vi "Teleop.vi"(10 "Match Info":T1={"Autonomous Elapsed Seconds"=0.0, "TeleOp Elapsed Seconds"=0.0, "Disabled Elapsed Seconds"=0.0, "Visited Autonomous"=FALSE, "Visited TeleOp"=FALSE, "Visited Disabled"=FALSE, "Autonomous Settings"={"Autonomous Style"=enum."Independent", "VI Refnum"=refnum}}, 11 "Call Context":T2) -> ()   [LabVIEW 2017]
doc: "This VI is called for each enabled TeleOp packet received from the DS. It is typically used to read from joysticks and other inputs and update I/O or setpoints for timed control loops. It should complete and return within 20 milliseconds or risk missing DS packets."
uses:
  <vilib>/Rock Robotics/WPI/DriverStation/WPI_DriverStationDerivedRobotMode.ctl
  <vilib>/Rock Robotics/WPI/DriverStation/WPI_DriverStationMatch Info.ctl
  <vilib>/Rock Robotics/WPI/Utilities/WPI_GetSetVariantRefNum.vi
  <vilib>/Rock Robotics/Network Tables/NT Write Boolean Array.vi
  <vilib>/Rock Robotics/Network Tables/NT Write Numeric Array.vi
  Framework/Robot Global Data.vi
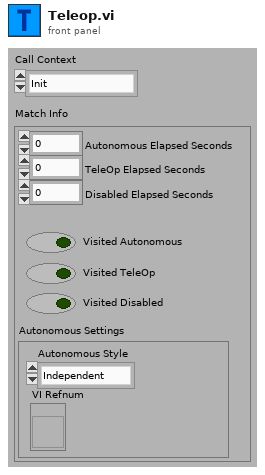
[diagram p1: front panel]
types:
  T1 = typedef "WPI_DriverStationMatch Info.ctl" = cluster{"Autonomous Elapsed Seconds":dbl, "TeleOp Elapsed Seconds":dbl, "Disabled Elapsed Seconds":dbl, "Visited Autonomous":bool, "Visited TeleOp":bool, "Visited Disabled":bool, "Autonomous Settings":cluster{"Autonomous Style":enum16{"Iterative", "Independent"}, "VI Refnum":refnum<vi>}}
  T2 = typedef "WPI_DriverStationDerivedRobotMode.ctl" = enum16{"Init", "Execute", "Stop"}
  T3 = enum16{"Linear", "Square  Root", "Square", "n^x"}
  T4 = typedef "WPI_JoystickDevRef.ctl" = cluster{"Device":T5}
  T5 = typedef "WPI_JoystickDeviceEnum.ctl" = enum16{"USB 0", "USB 1", "USB 2", "USB 3", "USB 4", "USB 5"}
  T6 = cluster{"X":dbl, "Y":dbl, "Angle":dbl, "Magnitude":dbl}
  T7 = typedef "Command Status Info.ctl" = cluster{"Name":string, "Status":T8, "notifier out":T9}
  T8 = typedef "Completion Status.ctl" = enum16{"Successful", "Aborted", "Incomplete"}
  T9 = typedef "Completion Notifier.ctl" = refnum<notifier>
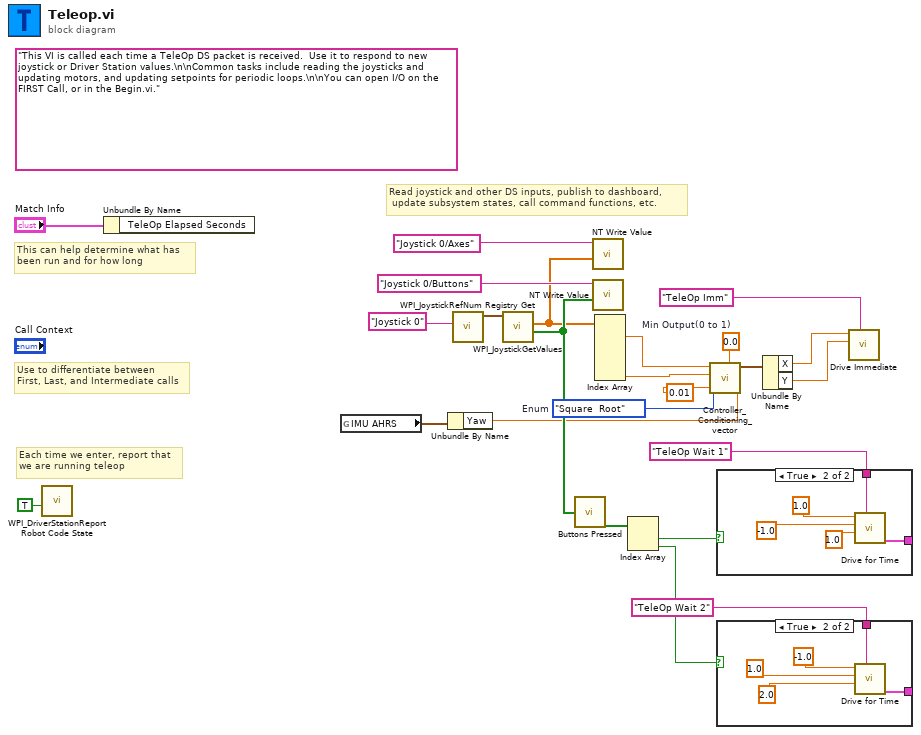
[diagram p0: block diagram]
diagram:
  w4 = T3."Square  Root"  # Enum
  w5 = 0.0  # Min Output(0 to 1)
  (unwired) "This VI is called each time a TeleOp DS packet is received.  Use it to respond to new joystick or Driver Station values.\n\nCommon tasks include reading the joysticks and updating motors, and updating setpoints for periodic loops.\n\nYou can open I/O on the FIRST Call, or in the Begin.vi."
  # "Read joystick and other DS inputs, publish to dashboard,\n update subsystem states, call command functions, etc."
  # "Each time we enter, report that\nwe are running teleop"
  # "Use to differentiate between\nFirst, Last, and Intermediate calls"
  # "This can help determine what has\nbeen run and for how long"
  n1 = call <vilib>:"WPI_DriverStationReport Robot Code State.vi"("TeleOp"=TRUE ("Autonomous")) -> ()  [unwired: 10 in, 1 out]
  n2 = Unbundle By Name("Match Info") -> ()  [unwired: 1 out]
  n3 = global read "Robot Global Data.vi" "IMU AHRS"() -> (w8:cluster{"Pitch":dbl, "Roll":dbl, "Yaw":dbl})
  n4 = Unbundle By Name(w8) -> ("Yaw"=w7:dbl)
  n5 = call <vilib>:"WPI_JoystickRefNum Registry Get.vi"("refnum name"="Joystick 0") -> ("JoystickDevRef"=w21:T4)  [unwired: 1 in, 9 out]
  n6 = call <vilib>:"WPI_JoystickGetValues.vi"("JoystickDevRef"=w21) -> ("Buttons"=w13:bool[], "Axes"=w12:dbl[])  [unwired: 6 in, 3 out]
  n7 = call "Buttons Pressed.vi"("Button Values"=w13) -> ("Button Presses"=w17:bool[])
  n8 = call-poly <vilib>:"NT Write Value.vi"("Numeric Array"=w12, "Name"="Joystick 0/Axes") -> ()  [unwired: 9 in, 1 out]
  n9 = call-poly <vilib>:"NT Write Value.vi"("Boolean Array"=w13, "Name"="Joystick 0/Buttons") -> ()  [unwired: 9 in, 1 out]
  n10 = Index Array(array=w12) -> (element #1=w10:dbl, element #6=w9:dbl)  [unwired: 6 in, 4 out]
  n11 = Index Array(array=w17) -> (element #1=w16:bool, element #2=w15:bool)  [unwired: 2 in]
  n12 = call "Controller_Conditioning_vector.vi"("Angular Offset\n(-180 to 180 or 0 to 360)"=w7, "Min Output(0 to 1)"=w5, "Enum"=w4, "Dead Zone(0 to 1)"=0.01, "Y(-1 to 1)"=w9, "X(-1 to 1)"=w10) -> ("output cluster"=w3:T6)  [unwired: 5 in]
  n13 = case shown="True" w16 {
    tunnel: [_ w28] -> _
    tunnel: "TeleOp Wait 1" ("Description") -> [_ w27]
    frame False {
    }
    frame True {
      n14 = call "Drive for Time.vi"("Description"=w27, "Seconds"=1.0, "Right Speed"=-1.0, "Left Speed"=1.0) -> ("Command Info Out"=w28:T7)  [unwired: 6 in, 1 out]
    }
  }
  n15 = case shown="True" w15 {
    tunnel: [_ w32] -> _
    tunnel: "TeleOp Wait 2" ("Description") -> [_ w31]
    frame False {
    }
    frame True {
      n16 = call "Drive for Time.vi"("Description"=w31, "Seconds"=2.0, "Right Speed"=1.0, "Left Speed"=-1.0) -> ("Command Info Out"=w32:T7)  [unwired: 6 in, 1 out]
    }
  }
  n17 = Unbundle By Name(w3) -> ("X"=w2:dbl, "Y"=w1:dbl)
  n18 = call "Drive Immediate.vi"("Description"="TeleOp Imm", "Right Setpoint"=w1, "Left Setpoint"=w2) -> ()  [unwired: 8 in, 1 out]
